vi "RPi HMI Global.vi"(7 "Mode":T1, 11 "HMI Cluster":T2={"Error"={"status"=FALSE, "code"=0, "source"=""}, "COM Ref"="", "Pump Data"={"Voltages"=[], "PumpCurrent"=[], "Speed"=[], "ControllerCurrent"=[], "Pressure"=[], "Flow"=[], "Elapsed Time (Display)"=[], "Avg Pressure"=0.0, "Avg Speed"=0.0, "Elapsed Time"=[4074.9003000000002, 4074.9003000000002, 4074.9003000000002, 4074.9003000000002, 4074.9003000000002, 4074.9003000000002]}, "Tank Data"={"PS Actual (V):"=0.0, "Temp1"=0.0, "Temp2"=0.0}, "Power Relays"={"Pump 1"=FALSE, "Pump 2"=FALSE, "Pump 3"=FALSE, "Pump 4"=FALSE, "Pump 5"=FALSE, "Pump 6"=FALSE}, "Pump CMDs"=[], "HMI Header"={"Line 1"="", "Line 2"="", "Line 3"="", "Line 4"=""}, "Tank CMDs"={"PS CMD"=0.0, "Press CMD"=0.0, "Temp 1 CMD"=0.0, "Temp 2 CMD"=0.0}, "HMI Tog Buttons"={"Start Test"=FALSE, "Toggle Spare 1"=FALSE, "Toggle Spare 2"=FALSE, "Toggle Spare 3"=FALSE, "Toggle Spare 4"=FALSE, "Toggle Spare 5"=FALSE}, "In Test"=FALSE, "HMI Command"=FALSE, "HMI Mom Buttons"={"Stop"=FALSE, "Reset Timers"=FALSE, "Log Fuel Change"=FALSE, "Alarm Dismiss"=FALSE}, "Controller Config"={"Controller Name"=enum."Kuhnke", "CommSeg"=0, "PWM?"=FALSE, "Frequency"=0, "Low Command"=0.0, "High Command"=0.0, "Stop Command"=0.0, "Command Step"=0.0, "Solenoid Stop?"=FALSE, "Controller?"=FALSE, "Invert PWM"=FALSE}, "Alarm"=FALSE, "Alarm Message 1"="", "Alarm Message 2"="", "Recording"=FALSE, "Serial Numbers"=[], "Pumps Present"=[]} {"Pump Data"."Elapsed Time" format="%<%H:%M:%S>t"; "Pump Data"."Elapsed Time (Display)" format="%<%H:%M:%S>t"; "Pump Data"."Speed" format="%#_4f"; "Pump Data"."ControllerCurrent" format="%#.1g"; "Pump Data"."Pressure" format="%#.0f"; "Pump Data"."Flow" format="%#.0f"; "Pump Data"."PumpCurrent" format="%#.1g"; "Pump Data"."Voltages" format="%#.0f"}) -> (3 "HMI Cluster OUT":T2={"Error"={"status"=FALSE, "code"=0, "source"=""}, "COM Ref"="", "Pump Data"={"Voltages"=[], "PumpCurrent"=[], "Speed"=[], "ControllerCurrent"=[], "Pressure"=[], "Flow"=[], "Elapsed Time (Display)"=[], "Avg Pressure"=0.0, "Avg Speed"=0.0, "Elapsed Time"=[4074.9003000000002, 4074.9003000000002, 4074.9003000000002, 4074.9003000000002, 4074.9003000000002, 4074.9003000000002]}, "Tank Data"={"PS Actual (V):"=0.0, "Temp1"=0.0, "Temp2"=0.0}, "Power Relays"={"Pump 1"=FALSE, "Pump 2"=FALSE, "Pump 3"=FALSE, "Pump 4"=FALSE, "Pump 5"=FALSE, "Pump 6"=FALSE}, "Pump CMDs"=[], "HMI Header"={"Line 1"="", "Line 2"="", "Line 3"="", "Line 4"=""}, "Tank CMDs"={"PS CMD"=0.0, "Press CMD"=0.0, "Temp 1 CMD"=0.0, "Temp 2 CMD"=0.0}, "HMI Tog Buttons"={"Start Test"=FALSE, "Toggle Spare 1"=FALSE, "Toggle Spare 2"=FALSE, "Toggle Spare 3"=FALSE, "Toggle Spare 4"=FALSE, "Toggle Spare 5"=FALSE}, "In Test"=FALSE, "HMI Command"=FALSE, "HMI Mom Buttons"={"Stop"=FALSE, "Reset Timers"=FALSE, "Log Fuel Change"=FALSE, "Alarm Dismiss"=FALSE}, "Controller Config"={"Controller Name"=enum."Kuhnke", "CommSeg"=0, "PWM?"=FALSE, "Frequency"=0, "Low Command"=0.0, "High Command"=0.0, "Stop Command"=0.0, "Command Step"=0.0, "Solenoid Stop?"=FALSE, "Controller?"=FALSE, "Invert PWM"=FALSE}, "Alarm"=FALSE, "Alarm Message 1"="", "Alarm Message 2"="", "Recording"=FALSE, "Serial Numbers"=[], "Pumps Present"=[]} {"Pump Data"."Elapsed Time" format="%<%H:%M:%S>t"; "Pump Data"."Elapsed Time (Display)" format="%<%H:%M:%S>t"; "Pump Data"."Speed" format="%#_4f"; "Pump Data"."ControllerCurrent" format="%#.1g"; "Pump Data"."Pressure" format="%#.0f"; "Pump Data"."Flow" format="%#.0f"; "Pump Data"."PumpCurrent" format="%#.1g"; "Pump Data"."Voltages" format="%#.0f"})   [LabVIEW 2018]
uses:
  Controls/HMI Cluster.ctl
  Controls/Pump Data.ctl
  Controls/HMI Header.ctl
  Controls/Tank CMDs.ctl
  Controls/HMI Tog Buttons.ctl
  Controls/HMI Mom Buttons.ctl
  Controls/Controller Config.ctl
  Type Defs/Controller Names.ctl
  Controls/HMI Global Mode.ctl
panel:
  in  "Power Relay":T10
  in  "Manual\nCMD":dbl[](array[numeric])=[0.0, 0.0, 0.0, 0.0, 0.0, 0.0] min=0.0 max=100.0 step=0.1 format="%#.2f"
  in  "Power Supply Cmd (V):":dbl min=0.0 max=20.0 format="%#.2f"
  in  "PressureCMD":dbl caption="Pressure Cmd (kPa):" min=0.0 max=825.0 format="%#.2f"
  in  "pb.Run Profile":bool
  in  "Tank 1 Setpoint":dbl caption="deg C"
  in  "Tank 2 Setpoint":dbl caption="deg C"
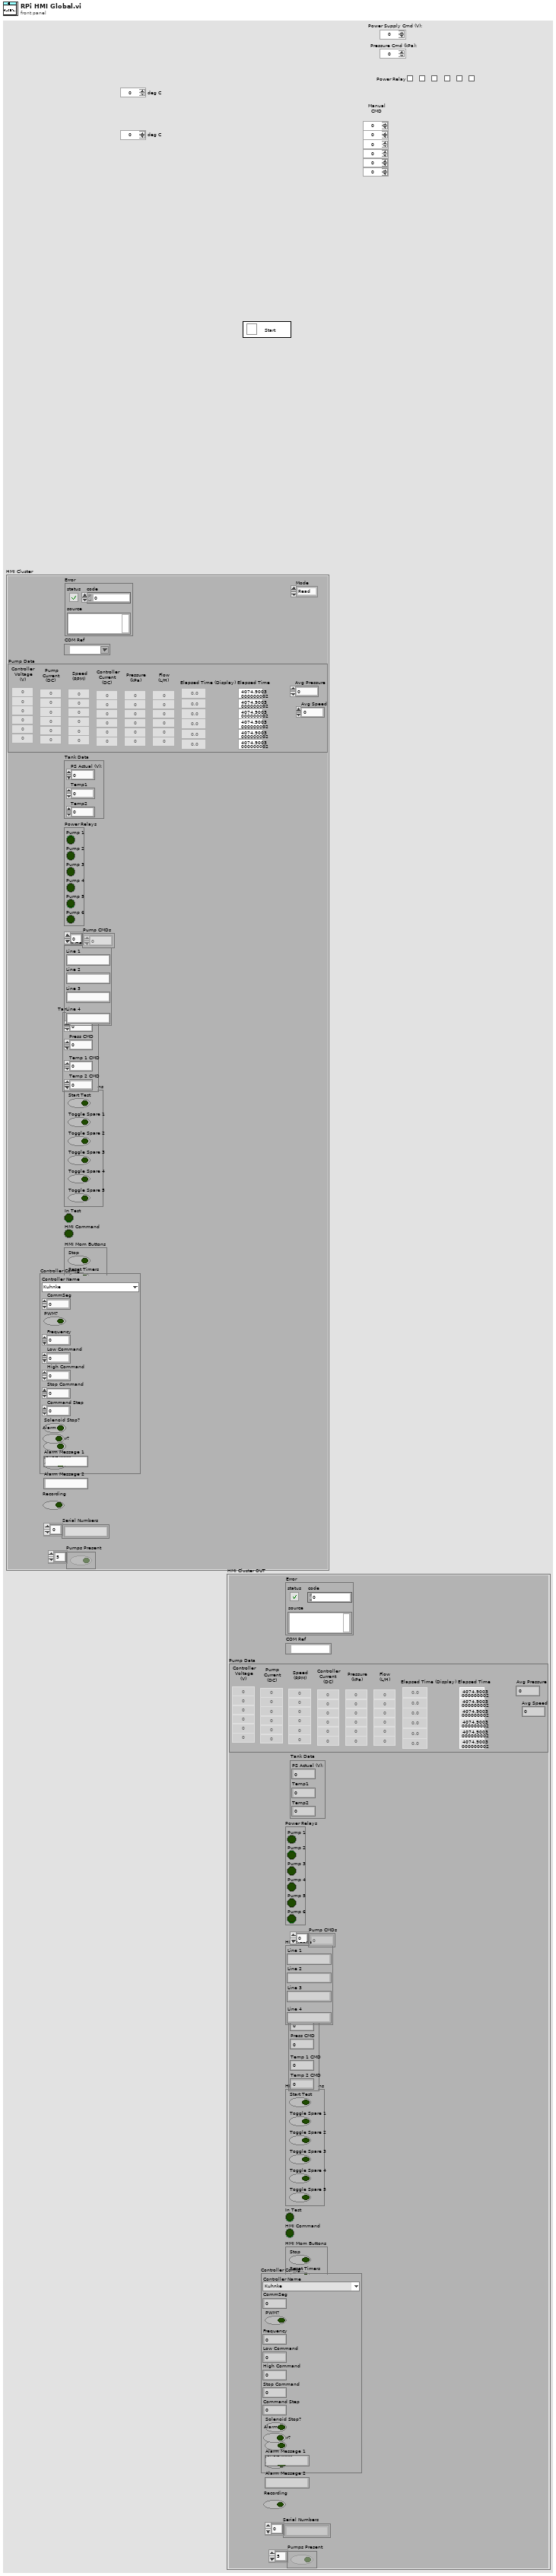
[diagram p1: front panel]
types:
  T1 = typedef "HMI Global Mode.ctl" = enum16{"Read", "Write Cluster", "Reset Cmd"}
  T2 = typedef "HMI Cluster.ctl" = cluster{"Error":errorcluster, "COM Ref":refnum<visa-resource-name>, "Pump Data":T3, "Tank Data":cluster{"PS Actual (V):":dbl, "Temp1":dbl, "Temp2":dbl}, "Power Relays":cluster{"Pump 1":bool, "Pump 2":bool, "Pump 3":bool, "Pump 4":bool, "Pump 5":bool, "Pump 6":bool}, "Pump CMDs":dbl[], "HMI Header":T4, "Tank CMDs":T5, "HMI Tog Buttons":T6, "In Test":bool, "HMI Command":bool, "HMI Mom Buttons":T7, "Controller Config":T8, "Alarm":bool, "Alarm Message 1":string, "Alarm Message 2":string, "Recording":bool, "Serial Numbers":string[], "Pumps Present":bool[]}
  T3 = typedef "Pump Data.ctl" = cluster{"Voltages":dbl[], "PumpCurrent":dbl[], "Speed":dbl[], "ControllerCurrent":dbl[], "Pressure":dbl[], "Flow":dbl[], "Elapsed Time (Display)":dbl[], "Avg Pressure":dbl, "Avg Speed":dbl, "Elapsed Time":dbl[]}
  T4 = typedef "HMI Header.ctl" = cluster{"Line 1":string, "Line 2":string, "Line 3":string, "Line 4":string}
  T5 = typedef "Tank CMDs.ctl" = cluster{"PS CMD":dbl, "Press CMD":dbl, "Temp 1 CMD":dbl, "Temp 2 CMD":dbl}
  T6 = typedef "HMI Tog Buttons.ctl" = cluster{"Start Test":bool, "Toggle Spare 1":bool, "Toggle Spare 2":bool, "Toggle Spare 3":bool, "Toggle Spare 4":bool, "Toggle Spare 5":bool}
  T7 = typedef "HMI Mom Buttons.ctl" = cluster{"Stop":bool, "Reset Timers":bool, "Log Fuel Change":bool, "Alarm Dismiss":bool}
  T8 = typedef "Controller Config.ctl" = cluster{"Controller Name":T9, "CommSeg":i32, "PWM?":bool, "Frequency":i32, "Low Command":dbl, "High Command":dbl, "Stop Command":dbl, "Command Step":dbl, "Solenoid Stop?":bool, "Controller?":bool, "Invert PWM":bool}
  T9 = typedef "Controller Names.ctl" = enum16{"Kuhnke", "Helbako BLDC", "Conti", "Hella BLDC OL PWM", "Hella BLDC Turbine OL PWM", "Hella BLDC Pressure", "Helbako (old)", "TI PWM", "PSA", "Hella Gas", "Hella Diesel", "8 Comm", "10 Comm", "8 Comm Hella", "10 Comm Hella", "8 Comm Omron", "10 Comm Omron", "8 Comm Nissan", "10 Comm Nissan"}
  T10 = cluster{"Pump 1":bool, "Pump 2":bool, "Pump 3":bool, "Pump 4":bool, "Pump 5":bool, "Pump 6":bool}
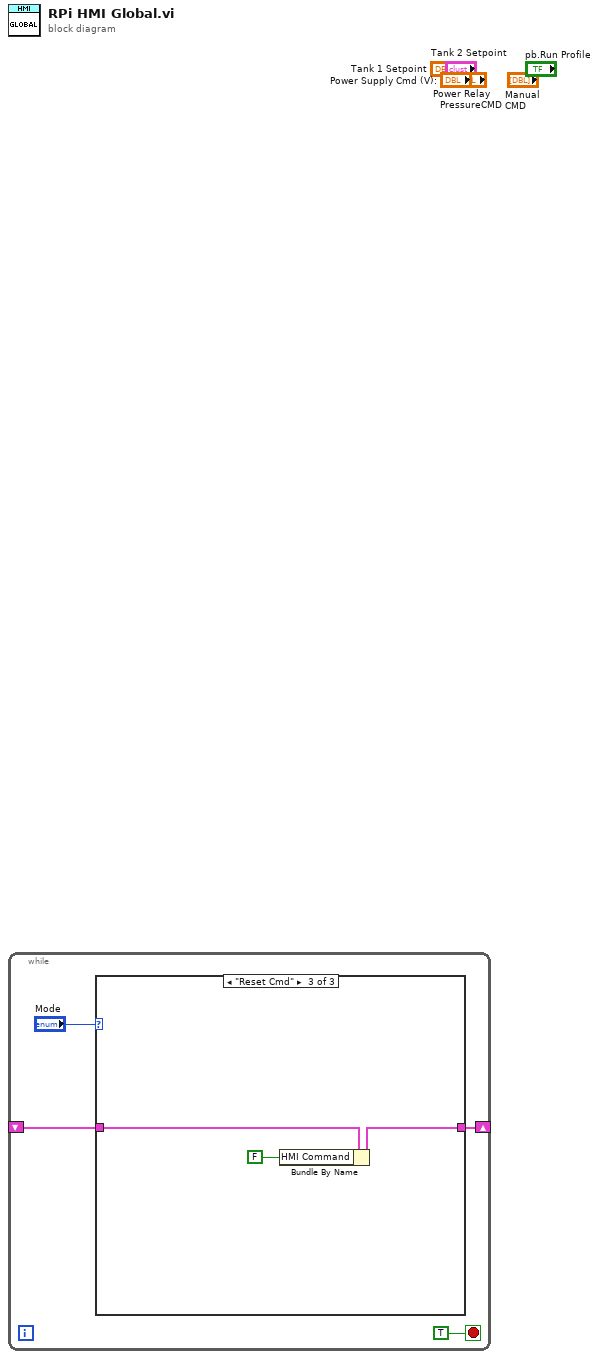
[diagram p0: block diagram]
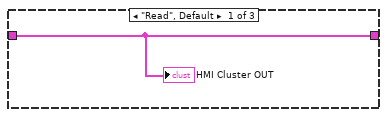
[diagram p2: hidden frame]
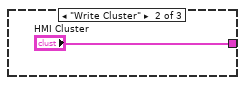
[diagram p3: hidden frame]
diagram:
  n1 = while {
    shift-right: [w3] -> _
    shift-left: _ -> [w2]
    stop <- TRUE stop-if-true
    n2 = case shown="\"Reset Cmd\"" "Mode" {
      tunnel: [w5 "HMI Cluster" w8] -> w3
      tunnel: w2 -> [w5 _ w9]
      frame "Read", Default {
        "HMI Cluster OUT" <- w5
      }
      frame "Write Cluster" {
      }
      frame "Reset Cmd" {
        n3 = Bundle By Name(cluster=w9, "HMI Command"=FALSE) -> (w8:T2)
      }
    }
  }
